vi "Combined Server.vi"   [LabVIEW 2015]
uses:
  CRDS/cCRDS/cCRDS.lvclass
  cPAS.lvclass
  Data/cPAS Data.lvclass
  Reusable/Session APIs/File Access/Config Data/Config Data.lvclass
  <vilib>/Platform/TimedLoop/XDataNode/timing_clust.ctl
  <vilib>/Platform/TimedLoop/XDataNode/nitl_modes.ctl
  <vilib>/Platform/TimedLoop/XDataNode/wakeup.ctl
  Reusable/Session APIs/File Access/Config Data/Config Data.lvclass/Config Data.ctl
  Devices/Alicat/Session Based/Data/Alicat Data.lvclass
  Reusable/Instrument/Instrument.lvclass/Instrument.ctl
  <vilib>/DAQmx/write.llb/DAQmx Write (Digital Bool 1Line 1Point).vi
  <vilib>/DAQmx/write.llb/DAQmx Write (Digital 1D Bool NChan 1Samp 1Line).vi
  Reusable/Instrument/Write Cfg Session.vi
  <vilib>/DAQmx/miscellaneous.llb/DAQmx Fill In Error Info.vi
  Write Serial IO.vi
  Reusable/PAS/Main/Write Data.vi
  CRDS/cCRDS/new/Data Access/Write SerialIO.vi
  <vilib>/Platform/TimedLoop/XDataNode/XDataNode.xnode
  Devices/CLAP/CLAP.lvclass
  Devices/Alicat/Session Based/Alicat Device.lvclass
  <userlib>/_Session Fwk/Session - Root.lvclass
  <vilib>/Platform/TimedLoop/XDataNode/XDNodeRunTimeDep.lvlib
types:
  T1 = typedef "Session - Root.lvclass/Session Handle.ctl" = refnum<data-value>
  T2 = typedef "XDNodeRunTimeDep.lvlib/timing_clust.ctl" = cluster{"Expected End [f-1]":u64, "Actual End [f-1]":u64, "Finished Late? [f-1]":bool, "Expected End [i-1]":u64, "Actual End [i-1]":u64, "Finished Late? [i-1]":bool, "Expected Start [i]":u64, "Actual Start [i]":u64, "Expected Start [f]":u64, "Actual Start [f]":u64, "Source Name":string, "Structure Name":string, "Period":i64, "Deadline":i64, "Offset":i64, "Start":i64, "Priority":i32, "Timeout":i32, "Mode":T3, "Wakeup Reason":T4, "Error":errorcluster, "Source Type":string, "Secondary Source Type":string, "Global End Time":u64, "Global Start Time":u64, "Frame Duration":u64, "Iteration Duration":u64, "Assigned CPU":i32, "I/O Scan Engine Mode":u32}
  T3 = typedef "XDNodeRunTimeDep.lvlib/nitl_modes.ctl" = enum32{"No Change", "Process missed periods, maintain original phase", "Discard missed periods, maintain original phase", "Process missed periods, ignore original phase", "Discard missed periods, ignore original phase"}
  T4 = typedef "XDNodeRunTimeDep.lvlib/wakeup.ctl" = enum32{"Normal", "Aborted", "Asynchronous wakeup", "Timing source error", "Timed loop error", "Timeout"}
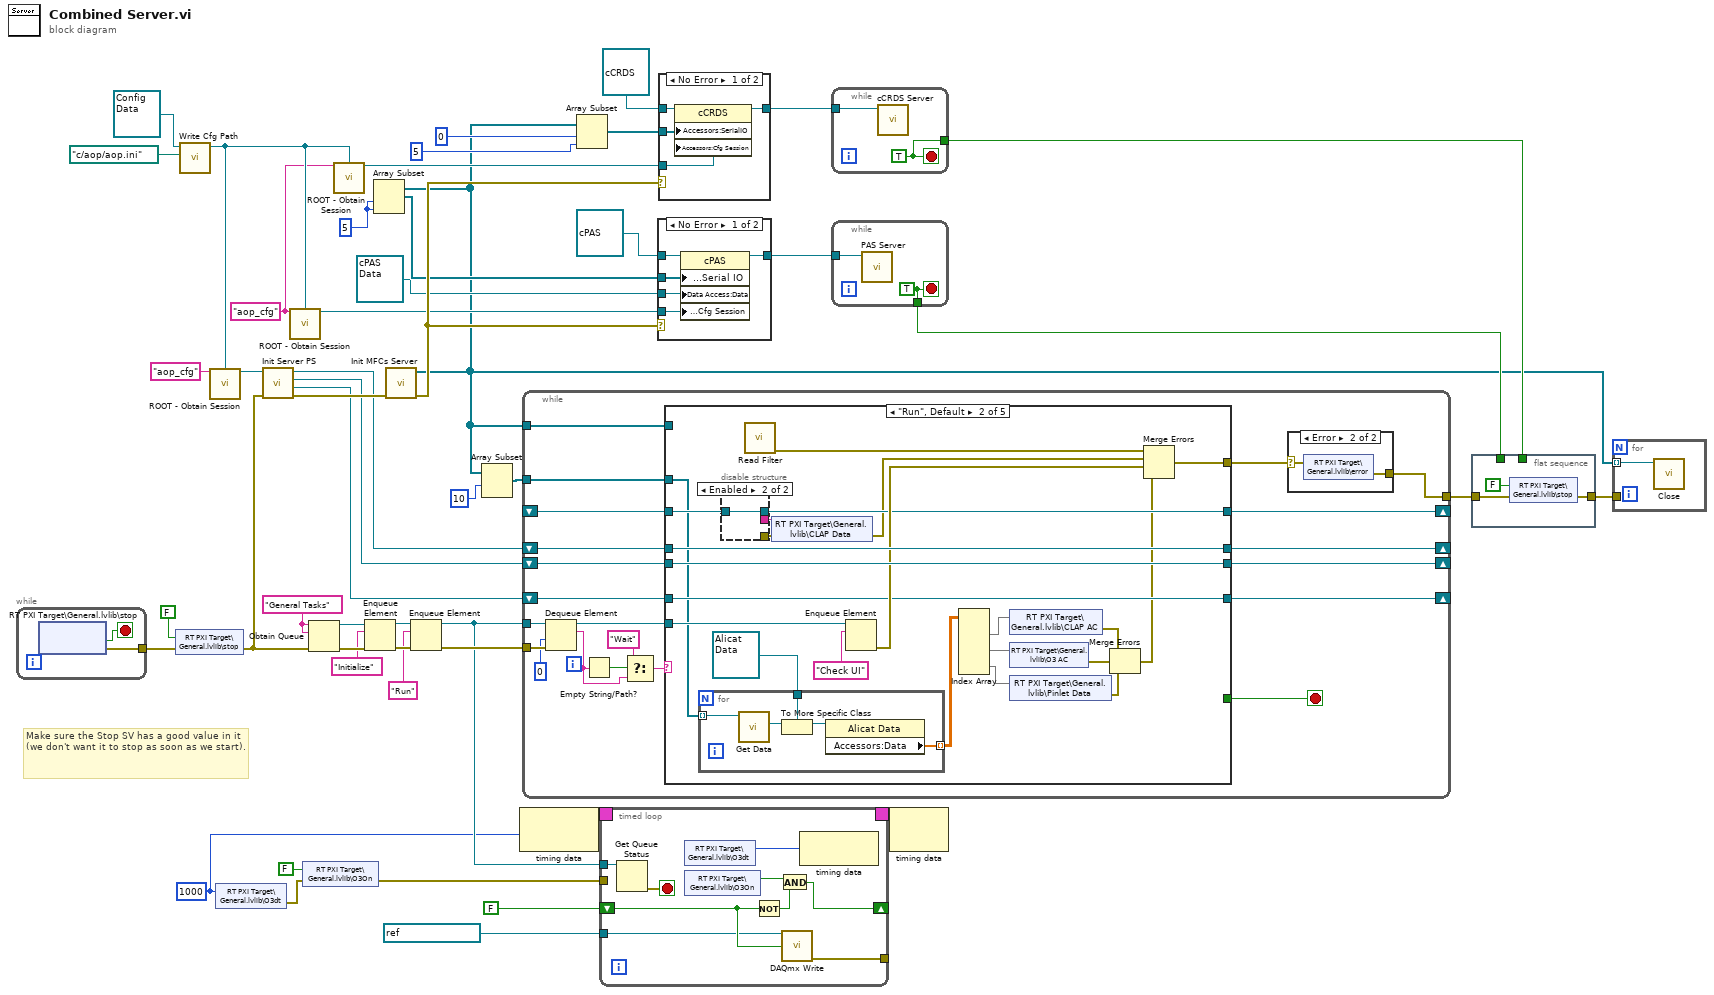
[diagram p0: block diagram]
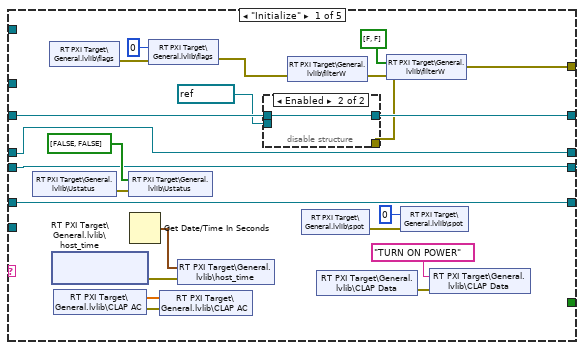
[diagram p3: hidden frame]
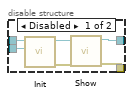
[diagram p4: hidden frame]
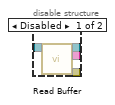
[diagram p5: hidden frame]
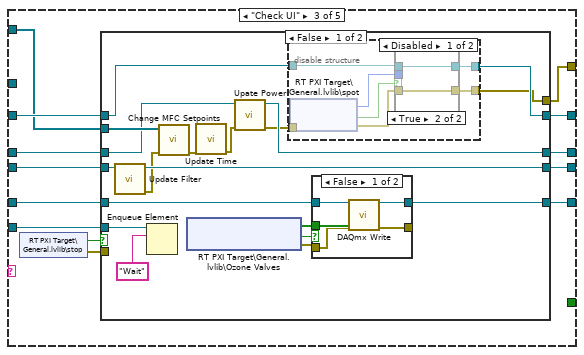
[diagram p6: hidden frame]
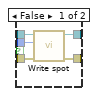
[diagram p7: hidden frame]
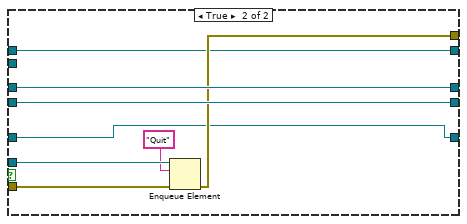
[diagram p10: hidden frame]
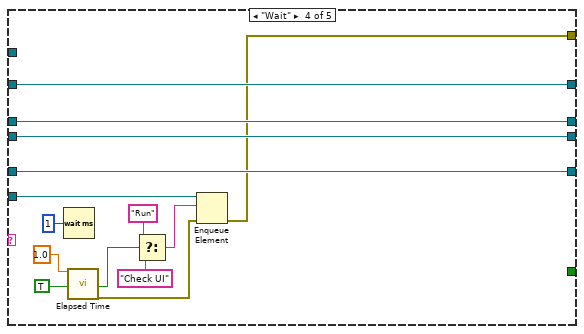
[diagram p11: hidden frame]
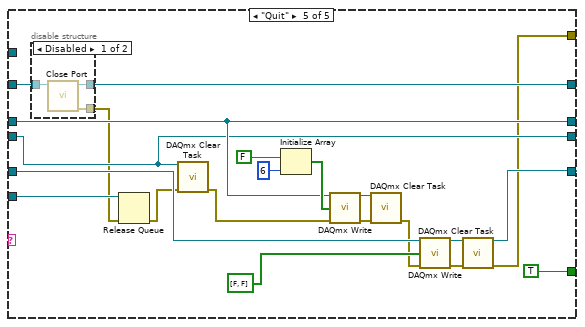
[diagram p12: hidden frame]
diagram:
  w4 = i64 1000 ("O3dt")
  w25 = "General Tasks" ("name (unnamed)")
  w11 = "aop_cfg" ("Session Name ()")
  w1 = 5 ("length")
  # "Make sure the Stop SV has a good value in it (we don't want it to stop as soon as we start)."
  n1 = while {
    tunnel: [w51] -> w49
    stop <- w52 stop-if-true
    n2 = shared-variable "RT PXI Target\\General.lvlib\\stop"() -> (error out=w51:errorcluster, w52:bool)  [unwired: 2 in, 1 out]
  }
  n3 = shared-variable "RT PXI Target\\General.lvlib\\stop"(FALSE ("stop"), error in=w49) -> (error out=w36:errorcluster)
  n4 = call "Write Cfg Path.vi"("Cfg Path"=path "c:/aop/aop.ini", "Config Data in"=refnum<class "Config Data.lvclass"> refnum ("Config Data")) -> ("Config Data out"=w13:refnum<class "Config Data.lvclass">)  [unwired: 8 in, 1 out]
  n5 = call <userlib>:"ROOT - Obtain Session.vi"("Session Name ()"="aop_cfg", "OBJ - Session"=w13) -> ("Session Handle"=w12:T1)  [unwired: 11 in, 2 out]
  n6 = shared-variable "RT PXI Target\\General.lvlib\\O3dt"(w4) -> (error out=w3:errorcluster)  [unwired: 1 in]
  n7 = call "Init Server PS.vi"("error in"=w36, "Cfg Handle"=w12) -> ("error out"=w42:errorcluster, "Ozone Out"=w39:refnum<k21>, "Filter Out Task"=w40:refnum<k21>, "PS Switch Out"=w41:refnum<k21>)  [unwired: 6 in]
  n8 = call <userlib>:"ROOT - Obtain Session.vi"("Session Name ()"=w11, "OBJ - Session"=w13) -> ("Session Handle"=w28:T1)  [unwired: 11 in, 2 out]
  n9 = shared-variable "RT PXI Target\\General.lvlib\\O3On"(FALSE ("O3On"), error in=w3) -> (error out=w2:errorcluster)
  n10 = Obtain Queue(name (unnamed)=w25, element data type=w25, error in (no error)=w36) -> (queue out=w24:refnum<queue>, error out=w23:errorcluster)  [unwired: 2 in, 1 out]
  n11 = call <userlib>:"ROOT - Obtain Session.vi"("Session Name ()"=w11, "OBJ - Session"=w13) -> ("Session Handle"=w27:T1)  [unwired: 11 in, 2 out]
  n12 = Enqueue Element(queue=w24, element="Initialize", error in (no error)=w23) -> (queue out=w21:refnum<queue>, error out=w20:errorcluster)  [unwired: 1 in, 1 out]
  n13 = call "Init MFCs Server.vi"("error in"=w42) -> ("error out"=w43:errorcluster, "Alicats"=w15:refnum<class "Alicat Device.lvclass">[])  [unwired: 9 in]
  n14 = Array Subset(array=w15, index=w1, length=w1) -> (w35:refnum<class "Alicat Device.lvclass">[])
  n15 = Enqueue Element(queue=w21, element="Run", error in (no error)=w20) -> (queue out=w8:refnum<queue>, error out=w19:errorcluster)  [unwired: 1 in, 1 out]
  n16 = Array Subset(array=w15, index=10) -> (w17:refnum<class "Alicat Device.lvclass">[])  [unwired: 1 in]
  n17 = node-c288(w4) -> (w10:T2)
  n18 = while {
    tunnel: w17 -> [w53]
    tunnel: w19 -> [w68]
    tunnel: w8 -> [w69]
    shift-right: [w70] -> _
    shift-left: w40 -> [w71]
    shift-right: [w72] -> _
    shift-left: w41 -> [w73]
    shift-right: [w63] -> _
    shift-left: _ -> [w62]
    tunnel: [w59] -> w48
    shift-right: [w57] -> _
    shift-left: w39 -> [w56]
    tunnel: w15 -> [w54]
    stop <- w61 stop-if-true
    n19 = Dequeue Element(queue=w69, timeout in ms (-1)=0, error in (no error)=w68) -> (queue out=w64:refnum<queue>, element=w66:string)  [unwired: 2 out]
    n20 = Empty String/Path?(string/path=w66) -> (empty?=w67:bool)
    n21 = Select(t="Wait", s=w67, f=w66) -> (s? t:f=w58:string)
    n22 = case shown="\"Run\", Default" w58 {
      tunnel: [w81 w123 w144 w201 w215] -> w55
      tunnel: w73 -> [w84 w126 w149 w213 w227]
      tunnel: [w84 w126 w147 w213 w227] -> w72
      tunnel: w53 -> [_ w112 _ _ _]
      tunnel: w71 -> [w83 w125 w151 w212 w226]
      tunnel: [w83 w125 w150 w212 w226] -> w70
      tunnel: w64 -> [_ w128 w148 w211 w224]
      tunnel: [w85 w120 w145 w214 w233] -> w63
      tunnel: w62 -> [w98 w121 w146 w214 w234]
      tunnel: [_ _ _ _ TRUE] -> w61
      tunnel: [w82 w118 w141 w210 w221] -> w57
      tunnel: w56 -> [w82 w118 w140 w210 w223]
      tunnel: w54 -> [_ _ w139 _ _]
      frame "Initialize" {
        n23 = shared-variable "RT PXI Target\\General.lvlib\\Ustatus"() -> (error out=w96:errorcluster)  [unwired: 1 in, 1 out]
        n24 = shared-variable "RT PXI Target\\General.lvlib\\flags"() -> (error out=w93:errorcluster)  [unwired: 1 in, 1 out]
        n25 = shared-variable "RT PXI Target\\General.lvlib\\host_time"() -> (error out=w94:errorcluster)  [unwired: 2 in, 2 out]
        n26 = shared-variable "RT PXI Target\\General.lvlib\\CLAP AC"() -> (w87:sgl[], error out=w88:errorcluster)  [unwired: 1 in]
        n27 = shared-variable "RT PXI Target\\General.lvlib\\Ustatus"(bool[] [FALSE, FALSE], error in=w96) -> ()  [unwired: 1 out]
        n28 = Get Date/Time In Seconds() -> (seconds since 1Jan1904=w95:timestamp)
        n29 = shared-variable "RT PXI Target\\General.lvlib\\flags"(u8 0 ("flags"), error in=w93) -> (error out=w80:errorcluster)
        n30 = shared-variable "RT PXI Target\\General.lvlib\\CLAP AC"(w87, error in=w88) -> ()  [unwired: 1 out]
        n31 = shared-variable "RT PXI Target\\General.lvlib\\host_time"(w95, error in=w94) -> ()  [unwired: 1 out]
        n32 = disable-structure shown="Enabled" {
          disable-tunnel: w98 -> [w104 w105]
          disable-tunnel: [w103 w105] -> w85
          disable-tunnel: [w102 _] -> w81
          disable-tunnel: refnum<visa-resource-name> "CLAP" ("Port") -> [w101 _]
          frame Disabled {
            n33 = call-dynamic "Init.vi"("Port"=w101, "CLAP in"=w104) -> ("error out"=w99:errorcluster, "CLAP out"=w100:refnum<class "CLAP.lvclass">)  [unwired: 8 in]
            n34 = call "Show.vi"("error in"=w99, "CLAP in"=w100) -> ("error out"=w102:errorcluster, "CLAP out"=w103:refnum<class "CLAP.lvclass">)  [unwired: 8 in]
          }
          frame Enabled {
          }
        }
        n35 = shared-variable "RT PXI Target\\General.lvlib\\filterW"(error in=w80) -> (error out=w92:errorcluster)  [unwired: 1 out]
        n36 = shared-variable "RT PXI Target\\General.lvlib\\spot"() -> (error out=w79:errorcluster)  [unwired: 1 in, 1 out]
        n37 = shared-variable "RT PXI Target\\General.lvlib\\CLAP Data"() -> (error out=w90:errorcluster)  [unwired: 1 in, 1 out]
        n38 = shared-variable "RT PXI Target\\General.lvlib\\filterW"(bool[] [FALSE, FALSE] ("filterW"), error in=w92) -> ()  [unwired: 1 out]
        n39 = shared-variable "RT PXI Target\\General.lvlib\\spot"(u8 0 ("spot"), error in=w79) -> ()  [unwired: 1 out]
        n40 = shared-variable "RT PXI Target\\General.lvlib\\CLAP Data"("TURN ON POWER" ("CLAP Data"), error in=w90) -> ()  [unwired: 1 out]
      }
      frame "Run", Default {
        n41 = for {
          tunnel: w112 -> [w133] mode=indexing
          tunnel: refnum<class "Alicat Data.lvclass"> refnum ("Alicat Data") -> [w131]
          tunnel: [w129] -> w110 mode=indexing
          n42 = call-dynamic "Get Data.vi"("Cfg Dev in"=w133) -> ("DataOut"=w132:refnum<class "Data.lvclass">)  [unwired: 8 in, 2 out]
          n43 = To More Specific Class(target class=w131, reference=w132) -> (specific class reference=w130:refnum<class "Alicat Data.lvclass">)  [unwired: 1 in, 1 out]
          n44 = property class="Alicat Data"(reference=w130) -> ("Accessors:Data"=w129:sgl[])  [unwired: 1 in, 2 out]
        }
        n45 = disable-structure shown="Enabled" {
          disable-tunnel: w121 -> [w137 w138]
          disable-tunnel: [w136 w138] -> w120
          disable-tunnel: [w135 _] -> w114
          disable-tunnel: [w134 _] -> w113
          frame Disabled {
            n46 = call "Read Buffer.vi"("CLAP in"=w137) -> ("error out"=w134:errorcluster, "Buffer"=w135:string, "CLAP out"=w136:refnum<class "CLAP.lvclass">)  [unwired: 8 in]
          }
          frame Enabled {
          }
        }
        n47 = call "Read Filter.vi"() -> ("error out"=w124:errorcluster)  [unwired: 11 in]
        n48 = shared-variable "RT PXI Target\\General.lvlib\\CLAP Data"(w114, error in=w113) -> (error out=w119:errorcluster)
        n49 = Enqueue Element(queue=w128, element="Check UI") -> (error out=w122:errorcluster)  [unwired: 2 in, 2 out]
        n50 = Index Array(array=w110) -> (element #1=w109:sgl[], element #2=w108:sgl[], element #3=w107:sgl[])  [unwired: 6 in]
        n51 = shared-variable "RT PXI Target\\General.lvlib\\CLAP AC"(w109) -> (error out=w117:errorcluster)  [unwired: 1 in]
        n52 = shared-variable "RT PXI Target\\General.lvlib\\O3 AC"(w108) -> (error out=w116:errorcluster)  [unwired: 1 in]
        n53 = shared-variable "RT PXI Target\\General.lvlib\\Pinlet Data"(w107) -> (error out=w115:errorcluster)  [unwired: 1 in]
        n54 = Merge Errors(w117, w116, w115) -> (w106:errorcluster)
        n55 = Merge Errors(w124, w119, w122, w106) -> (w123:errorcluster)
      }
      frame "Check UI" {
        n56 = shared-variable "RT PXI Target\\General.lvlib\\stop"() -> (w142:bool, error out=w143:errorcluster)  [unwired: 1 in]
        n57 = case shown="False" w142 {
          tunnel: w151 -> [w170 w197]
          tunnel: [w169 w197] -> w150
          tunnel: w139 -> [w168 _]
          tunnel: w149 -> [w167 w198]
          tunnel: w148 -> [w153 w200]
          tunnel: [w166 w198] -> w147
          tunnel: w146 -> [w165 w194]
          tunnel: [w164 w194] -> w145
          tunnel: [w163 w195] -> w144
          tunnel: w143 -> [_ w196]
          tunnel: [w156 w193] -> w141
          tunnel: w140 -> [w157 w193]
          frame False {
            n58 = call "Update Filter.vi"("Refnum in"=w170) -> ("error out"=w162:errorcluster, "Refnum out"=w169:refnum<k21>)  [unwired: 9 in]
            n59 = Enqueue Element(queue=w153, element="Wait") -> ()  [unwired: 2 in, 3 out]
            n60 = call "Change MFC Setpoints.vi"("error in"=w162, "Alicats"=w168) -> ("error out"=w161:errorcluster)  [unwired: 9 in]
            n61 = shared-variable "RT PXI Target\\General.lvlib\\Ozone Valves"() -> (w155:bool[], error out=w154:errorcluster, w158:bool)  [unwired: 2 in]
            n62 = call "Update Time.vi"("error in"=w161) -> ("error out"=w160:errorcluster)  [unwired: 10 in]
            n63 = call "Upate Power.vi"("error in"=w160, "Refnum in"=w167) -> ("error out"=w159:errorcluster, "Refnum out"=w166:refnum<k21>)  [unwired: 8 in]
            n64 = disable-structure shown="Disabled" {
              disable-tunnel: w165 -> [w177 w186]
              disable-tunnel: [w176 w186] -> w164
              disable-tunnel: [w175 w185] -> w163
              disable-tunnel: w159 -> [w174 w185]
              frame Disabled {
                n65 = shared-variable "RT PXI Target\\General.lvlib\\spot"(error in=w174) -> (w172:u8, error out=w173:errorcluster, w171:bool)  [unwired: 1 in]
                n66 = case shown="True" w171 {
                  tunnel: w177 -> [w182 w183]
                  tunnel: [w181 w183] -> w176
                  tunnel: [w180 w184] -> w175
                  tunnel: w173 -> [w179 w184]
                  tunnel: w172 -> [w178 _]
                  frame False {
                    n67 = call-dynamic "Write spot.vi"("error in"=w179, "spot"=w178, "CLAP in"=w182) -> ("error out"=w180:errorcluster, "CLAP out"=w181:refnum<class "CLAP.lvclass">)  [unwired: 7 in]
                  }
                  frame True {
                  }
                }
              }
              frame Enabled {
              }
            }
            n68 = case shown="False" w158 {
              tunnel: w157 -> [w191 w192]
              tunnel: [w190 w192] -> w156
              tunnel: w155 -> [w189 _]
              tunnel: w154 -> [w188 _]
              tunnel: [w187 _] -> _
              frame False {
                n69 = call-poly <vilib>:"DAQmx Write.vi"("task/channels in"=w191, "data"=w189, "error in"=w188) -> ("task out"=w190:refnum<k21>, "error out"=w187:errorcluster)  [unwired: 10 in, 1 out]
              }
              frame True {
              }
            }
          }
          frame True {
            n70 = Enqueue Element(queue=w200, element="Quit", error in (no error)=w196) -> (error out=w195:errorcluster)  [unwired: 1 in, 2 out]
          }
        }
      }
      frame "Wait" {
        n71 = Wait (ms)(milliseconds to wait=u32 1) -> ()  [unwired: 1 out]
        n72 = call "Elapsed Time"("Time Target (s)"=1.0, "Auto Reset"=TRUE) -> ("Time has Elapsed"=w206:bool, "error out"=w202:errorcluster)  [unwired: 10 in, 6 out]
        n73 = Select(t="Run" ("element"), s=w206, f="Check UI") -> (s? t:f=w203:string)
        n74 = Enqueue Element(queue=w211, element=w203, error in (no error)=w202) -> (error out=w201:errorcluster)  [unwired: 1 in, 2 out]
      }
      frame "Quit" {
        n75 = disable-structure shown="Disabled" {
          disable-tunnel: w234 -> [w237 _]
          disable-tunnel: [w236 _] -> w233
          disable-tunnel: [w235 _] -> w216
          frame Disabled {
            n76 = call-dynamic "Close Port.vi"("CLAP in"=w237) -> ("error out"=w235:errorcluster, "CLAP out"=w236:refnum<class "CLAP.lvclass">)  [unwired: 9 in]
          }
          frame Enabled {
          }
        }
        n77 = Release Queue(queue=w224, error in (no error)=w216) -> (error out=w219:errorcluster)  [unwired: 1 in, 2 out]
        n78 = call <vilib>:"DAQmx Clear Task.vi"("task in"=w226, "error in"=w219) -> ("error out"=w218:errorcluster)  [unwired: 13 in]
        n79 = Initialize Array(FALSE, 6 ("dimension size")) -> (w230:bool[])
        n80 = call-poly <vilib>:"DAQmx Write.vi"("task/channels in"=w227, "data"=w230, "error in"=w218) -> ("task out"=w231:refnum<k21>, "error out"=w232:errorcluster)  [unwired: 10 in, 1 out]
        n81 = call <vilib>:"DAQmx Clear Task.vi"("task in"=w231, "error in"=w232) -> ("error out"=w217:errorcluster)  [unwired: 13 in]
        n82 = call-poly <vilib>:"DAQmx Write.vi"("task/channels in"=w223, "data"=bool[] [FALSE, FALSE], "error in"=w217) -> ("task out"=w221:refnum<k21>, "error out"=w222:errorcluster)  [unwired: 10 in, 1 out]
        n83 = call <vilib>:"DAQmx Clear Task.vi"("task in"=w221, "error in"=w222) -> ("error out"=w215:errorcluster)  [unwired: 13 in]
      }
    }
    n84 = case shown="Error" w55 {
      selector: w55 -> [w74 w75]
      tunnel: [w74 w76] -> w59
      frame No Error {
      }
      frame Error {
        n85 = shared-variable "RT PXI Target\\General.lvlib\\error"(w75) -> (error out=w76:errorcluster)  [unwired: 1 in]
      }
    }
  }
  n86 = Array Subset(array=w15, index=0, length=5) -> (w32:refnum<class "Alicat Device.lvclass">[])
  n87 = timed-loop {
    timing: w10 -> [_]
    timing-out: [_] -> w9
    tunnel: w8 -> [w246]
    shift-right: [w241] -> _
    shift-left: FALSE -> [w243]
    tunnel: refnum<k21> "O3 Gen Level" ("task/channels in") -> [w239]
    tunnel: w2 -> [_]
    tunnel: [w238] -> _
    stop <- w245 stop-if-true
    n88 = Get Queue Status(queue=w246) -> (error out=w245:errorcluster)  [unwired: 2 in, 7 out]
    n89 = shared-variable "RT PXI Target\\General.lvlib\\O3dt"() -> (w240:i64)  [unwired: 1 in, 1 out]
    n90 = shared-variable "RT PXI Target\\General.lvlib\\O3On"() -> (w244:bool)  [unwired: 1 in, 1 out]
    n91 = Not(x=w243) -> (.not. x?=w242:bool)
    n92 = And(x=w244, y=w242) -> (x .and. y?=w241:bool)
    n93 = call-poly <vilib>:"DAQmx Write.vi"("task/channels in"=w239, "data"=w243) -> ("error out"=w238:errorcluster)  [unwired: 11 in, 2 out]
    n94 = node-c288(w240) -> ()  [unwired: 1 out]
  }
  n95 = case shown="No Error" w43 {
    tunnel: refnum<class "cPAS.lvclass"> refnum ("cPAS") -> [w255 w256]
    tunnel: [w254 w256] -> w45
    tunnel: w35 -> [w253 _]
    tunnel: refnum<class "cPAS Data.lvclass"> refnum ("cPAS Data") -> [w252 _]
    tunnel: w28 -> [w251 _]
    frame No Error {
      n96 = property class="cPAS"(reference=w255, "Data Access:Serial IO"=w253, "Data Access:Data"=w252, "Accessors:Cfg Session"=w251) -> (reference out=w254:refnum<class "cPAS.lvclass">)  [unwired: 1 in, 1 out]
    }
    frame Error {
    }
  }
  n97 = case shown="No Error" w43 {
    tunnel: refnum<class "cCRDS.lvclass"> refnum ("cCRDS") -> [w260 w261]
    tunnel: [w259 w261] -> w44
    tunnel: w32 -> [w258 _]
    tunnel: w27 -> [w257 _]
    frame No Error {
      n98 = property class="cCRDS"(reference=w260, "Accessors:SerialIO"=w258, "Accessors:Cfg Session"=w257) -> (reference out=w259:refnum<class "cCRDS.lvclass">)  [unwired: 1 in, 1 out]
    }
    frame Error {
    }
  }
  n99 = while {
    tunnel: w44 -> [w263]
    tunnel: [w262] -> w37
    stop <- w262 stop-if-true
    w262 = TRUE
    n100 = call "cCRDS Server.vi"("cCRDS"=w263) -> ()  [unwired: 11 in]
  }
  n101 = while {
    tunnel: w45 -> [w265]
    tunnel: [w264] -> w38
    stop <- w264 stop-if-true
    w264 = TRUE
    n102 = call "PAS Server.vi"("PASIn"=w265) -> ()  [unwired: 11 in]
  }
  n103 = node-c288(w9) -> ()  [unwired: 1 out]
  n104 = flat-sequence {
    tunnel: w48 -> [w267]
    tunnel: [w266] -> w26
    tunnel: w38 -> [_]
    tunnel: w37 -> [_]
    frame #0 {
      n105 = shared-variable "RT PXI Target\\General.lvlib\\stop"(FALSE ("stop"), error in=w267) -> (error out=w266:errorcluster)
    }
  }
  n106 = for {
    tunnel: w15 -> [w269] mode=indexing
    tunnel: w26 -> [_]
    n107 = call-dynamic "Close.vi"("Cfg Dev in"=w269) -> ()  [unwired: 9 in, 2 out]
  }
